vi "Set DC Voltage.vi"(8 "error in (no error)":errorcluster, 10 "Output Voltage [V]":dbl format="%.4f", 11 "VISA name":refnum<visa-resource-name>="GPIB::5::INSTR") -> (0 "error out":errorcluster)   [LabVIEW 2020, in "Low Level PSU With Tests.lvlib"]
uses:
  VISA/VISA Instrument.lvclass
  C:/Git/astemes-gdevcon-2022/PSU Demo/Low Level PSU With Tests/Instrument Interface/Instrument.lvclass
  Low Level PSU With Tests.lvlib
  Low Level PSU/Low Level PSU.lvclass
  C:/Git/astemes-gdevcon-2022/PSU Demo/Low Level PSU With Tests/VISA/VISA Instrument.lvclass
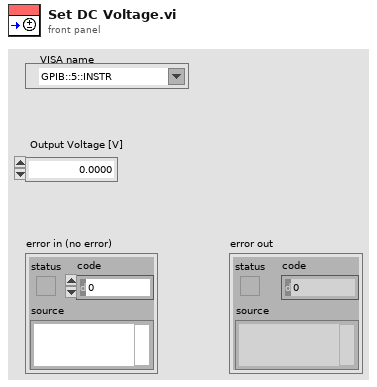
[diagram p1: front panel]
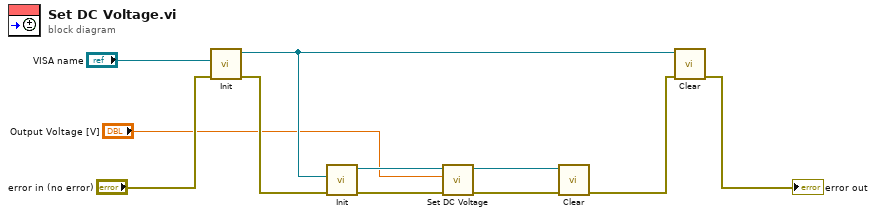
[diagram p0: block diagram]
diagram:
  n1 = call "Init.vi"("error in (no error)"="error in (no error)", "VISA name"="VISA name") -> ("error out"=w8:errorcluster, "VISA out"=w4:refnum<class "VISA Instrument.lvclass">)  [unwired: 8 in]
  n2 = call "Init.vi"("error in (no error)"=w8, "Instrument Interface"=w4) -> ("error out"=w11:errorcluster, "Low Level PSU Out"=w3:refnum<class "Low Level PSU.lvclass">)  [unwired: 8 in]
  n3 = call "Set DC Voltage.vi"("error in (no error)"=w11, "Volt"="Output Voltage [V]", "Low Level PSU in"=w3) -> ("error out"=w10:errorcluster, "Low Level PSU out"=w2:refnum<class "Low Level PSU.lvclass">)  [unwired: 7 in]
  n4 = call "Clear.vi"("error in (no error)"=w10, "Low Level PSU In"=w2) -> ("error out"=w7:errorcluster)  [unwired: 8 in, 1 out]
  n5 = call "Clear.vi"("error in (no error)"=w7, "VISA in"=w4) -> ("error out"=→"error out":errorcluster)  [unwired: 8 in, 1 out]
